vi "hardware status globals.vi"() -> ()   [LabVIEW 2016]
uses:
  shutters status.ctl
  new-h-nu-ixon/Laser type.ctt
  new-h-nu-ixon/Emission filters.ctl
panel:
  in  "Emission filter status":T1
  out "Camera status":bool
  in  "Shutters Status":T2=[{"Laser"=enum."Blue 488 nm", "Status"=FALSE}, {"Laser"=enum."Green 532 nm", "Status"=FALSE}, {"Laser"=enum."Red 635 nm", "Status"=FALSE}, {"Laser"=enum."IR 785", "Status"=FALSE}]
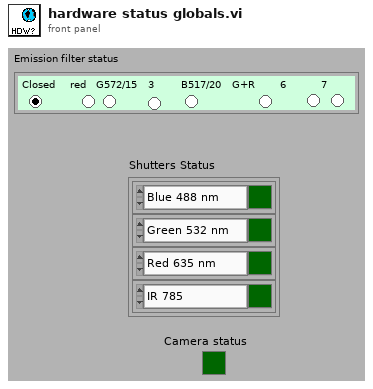
[diagram p1: front panel]
types:
  T1 = typedef "Emission filters.ctl" = enum32{" Closed ", " red ", "G572/15", "3", "B517/20", "G+R", "6", "7"}
  T2 = typedef "shutters status.ctl" = cluster{"Laser":T3, "Status":bool}[]
  T3 = typedef "Laser type.ctt" = enum16{"Blue 488 nm", "Green 532 nm", "Red 635 nm", "IR 785"}
diagram:
